vi "LINX - Blink (Simple).vi"() -> ()   [LabVIEW 2020]
doc: "Manually blink and LED attached to a digital output channel of a LINX device by clicking and LED control in LabVIEW."
uses:
  vi.lib/MakerHub/LINX/Public/Peripherals/Digital/Digital Write 1 Chan.vi
  vi.lib/MakerHub/LINX/Public/Peripherals/Digital/Digital Write N Chans.vi
  vi.lib/MakerHub/LINX/Private/Local IO/LinxDigitalWrite.vi
  vi.lib/MakerHub/LINX/Public/Utilities/Check Channel.vi
  vi.lib/MakerHub/LINX/Public/Utilities/Open Serial.vi
  vi.lib/MakerHub/LINX/Private/Utilties/Generate Error.vi
  vi.lib/MakerHub/LINX/LMH-LINX.lvlib
  vi.lib/MakerHub/LINX/Private/Device/Device.lvlib
panel:
  out "Loop Rate (Hz)":u32
  in  "LED Value":bool
  in  "Digital Output Channel":u8=13
  in  "Serial Port":refnum<visa-resource-name>
  in  "Stop Button":bool
  # "Circuit Schematic"
  # "LINX Device Settings"
  # "LED Control"
  # "Manual Blink Example\n\nThis example demonstrates how to blink an LED on a LINX device by clicking on an LED control in LabVIEW.\n\nInstructions\n1. Select the Serial Port associated with the LINX Device.\n2. Select the Digital Output Channel connected to the LED.\n3. Click the Run Arrow."
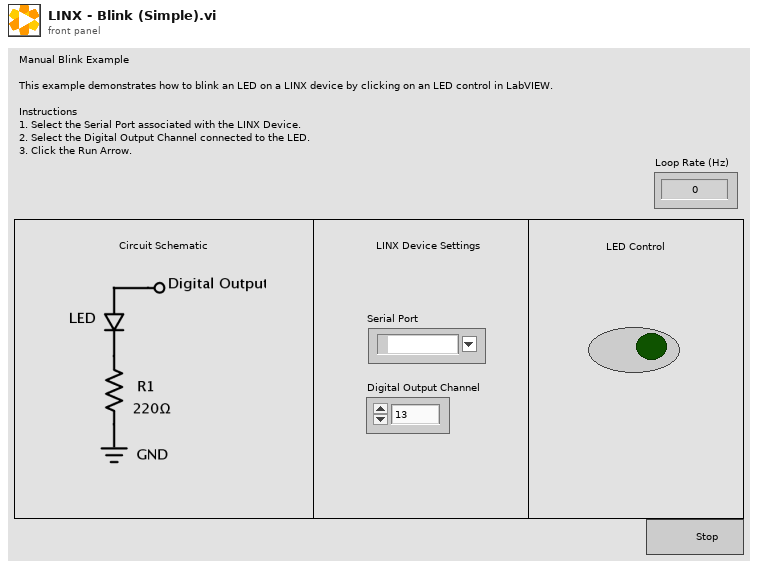
[diagram p1: front panel]
types:
  T1 = typedef "LMH-LINX.lvlib/LINX Ref.ctl" = cluster{"IO":T2, "Interface":T3, "LINX Device Config":T4}
  T2 = typedef "LMH-LINX.lvlib/Platform.ctl" = enum16{"Remote", "Local"}
  T3 = typedef "LMH-LINX.lvlib/Interface.ctl" = enum16{"Serial", "TCP"}
  T4 = typedef "Device.lvlib/LINX Device Config.ctl" = cluster{"Interface":T3, "COM Port":refnum<visa-resource-name>, "TCP Configuration":T5, "Device Family":u8, "Device ID":u8, "Device Name":string, "TCP Ref":refnum<k5>, "Channels":T6}
  T5 = typedef "Device.lvlib/TCP Config.ctl" = cluster{"IP Address":string, "Port":u16}
  T6 = typedef "LMH-LINX.lvlib/Channels.ctl" = cluster{"DI":u8[], "DO":u8[], "AI":u8[], "AO":u8[], "PWM":u8[], "QE":u8[], "UART":u8[], "I2C 2":u8[], "SPI":u8[], "CAN":u8[], "Servo":u8[], "AI Ref (V)":dbl, "AI Resolution (Bits)":u8, "AO Ref (V)":dbl, "AO Resolution (Bits)":u8}
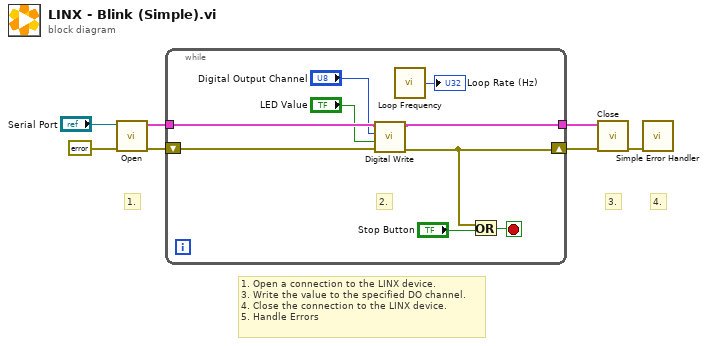
[diagram p0: block diagram]
diagram:
  # "1. Open a connection to the LINX device.\n3. Write the value to the specified DO channel.\n4. Close the connection to the LINX device.\n5. Handle Errors"
  # "4."
  # "3."
  # "1."
  n1 = call-poly "Open.vi"("Error In"=errorcluster {"status"=FALSE, "code"=0, "source"=""}, "Serial Port"="Serial Port") -> ("Error Out"=w6:errorcluster, "LINX Resource"=w7:T1)  [unwired: 7 in, 1 out]
  n2 = while {
    tunnel: w7 -> [w14]
    tunnel: [w13] -> w5
    shift-right: [w11] -> w4
    shift-left: w6 -> [w12]
    stop <- w16 stop-if-true
    # "2."
    n3 = call-poly "Digital Write.vi"("Error In"=w12, "Output Value"="LED Value", "DO Channel"="Digital Output Channel", "LINX Resource"=w14) -> ("Error Out"=w11:errorcluster, "LINX Resource"=w13:T1)  [unwired: 6 in]
    n4 = call "Loop Frequency.vi"() -> ("Loop Rate (Hz)"=→"Loop Rate (Hz)":u32)
    n5 = Or(x=w11, y="Stop Button") -> (x .or. y?=w16:bool)
  }
  n6 = call "Close.vi"("Error In"=w4, "LINX Resource"=w5) -> ("Error Out"=w2:errorcluster)  [unwired: 9 in]
  n7 = call <vilib>:"Simple Error Handler.vi"("error in (no error)"=w2) -> ()  [unwired: 4 in, 5 out]
